vi "testAggState.vi"(8 "error in (no error)":errorcluster) -> (0 "error out":errorcluster)   [LabVIEW 2016]
doc: "Test the aggState.vi."
uses:
  ZTAAC/ZTAAC.lvclass
  StrictDef/DofGroup.ctl
  StrictDef/InstName.ctl
  <vilib>/addons/_JKI Toolkits/Caraya/classes/Test/Test.lvclass
  <vilib>/addons/_JKI Toolkits/Caraya/classes/Assert/Assert.lvclass
panel:
  in  "ZTAAC.lvclass":refnum<class "ZTAAC.lvclass">
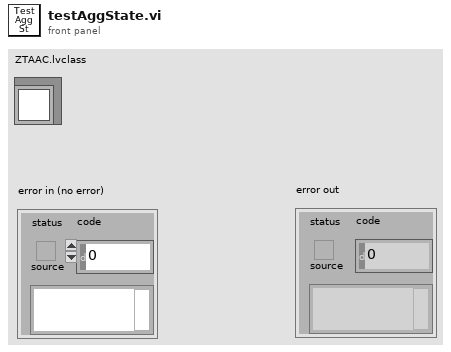
[diagram p1: front panel]
types:
  T1 = typedef "InstName.ctl" = enum16{"lsst", "comcam"}
  T2 = cluster{"Config Dir":path, "Inst Name":T1, "OptStateEsti Config File Name":string, "Mapping File Name":string, "Wavelength Table":string, "Intrinc Zk File Name":string, "y2 Corection File Name":string, "Index DOF File Name":string, "OptCtrl Config File Name":string, "State 0 File Name":string, "Weighting File Name":string, "PSSN Alpha File Name":string, "Authority Files":cluster{"Rigid Body Stroke File":string, "M1M3 Subsystem":cluster{"Mirror":string, "Actuatro Force File":string}, "M2 Subsystem":cluster{"Mirror":string, "Actuatro Force File":string}, "Num of Bending Mode":i32}, "Truncation Threshold":dbl}
  T3 = typedef "DofGroup.ctl" = enum16{"M2 Hex Pos", "Cam Hex Pos", "M1M3 Bend", "M2 Bend"}
  T4 = cluster{"M2 Hexapod":bool[], "Cam Hexapod ":bool[], "M1M3 Bending Mode":bool[], "M2 Bending Mode":bool[]}
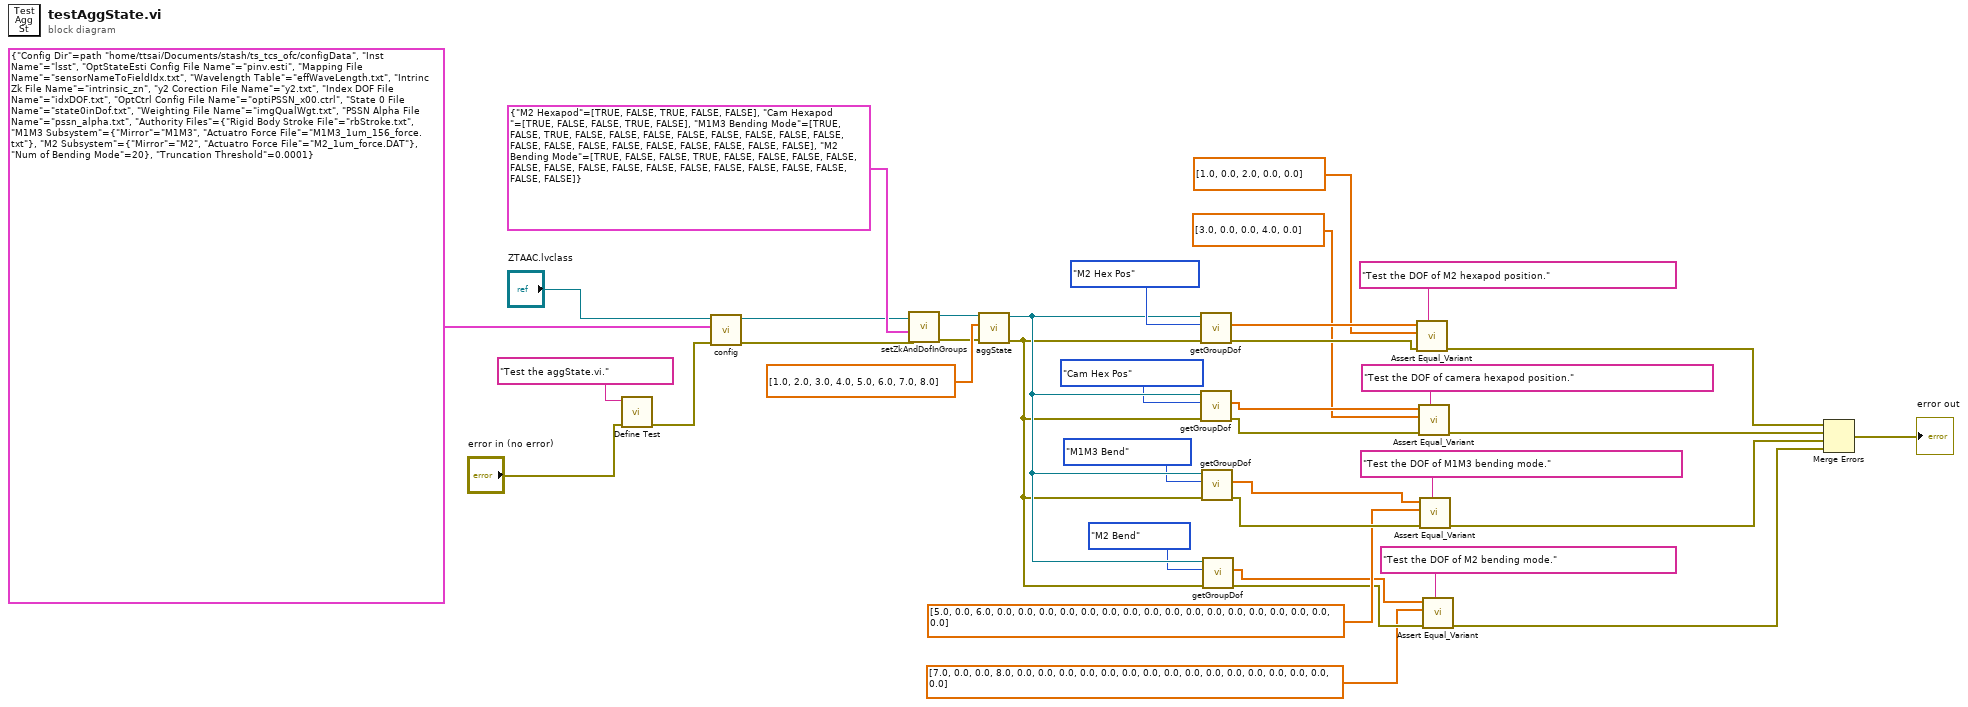
[diagram p0: block diagram]
diagram:
  n1 = call <vilib>:"Define Test.vi"("error in (no error)"="error in (no error)", "Label (VI Title)"="Test the aggState.vi.") -> ("error out"=w28:errorcluster)  [unwired: 9 in]
  n2 = call "config.vi"("error in (no error)"=w28, "ZTAAC Configuration"=T2 {"Config Dir"=path "/home/ttsai/Documents/stash/ts_tcs_ofc/configData", "Inst Name"=enum."lsst", "OptStateEsti Config File Name"="pinv.esti", "Mapping File Name"="sensorNameToFieldIdx.txt", "Wavelength Table"="effWaveLength.txt", "Intrinc Zk File Name"="intrinsic_zn", "y2 Corection File Name"="y2.txt", "Index DOF File Name"="idxDOF.txt", "OptCtrl Config File Name"="optiPSSN_x00.ctrl", "State 0 File Name"="state0inDof.txt", "Weighting File Name"="imgQualWgt.txt", "PSSN Alpha File Name"="pssn_alpha.txt", "Authority Files"={"Rigid Body Stroke File"="rbStroke.txt", "M1M3 Subsystem"={"Mirror"="M1M3", "Actuatro Force File"="M1M3_1um_156_force.txt"}, "M2 Subsystem"={"Mirror"="M2", "Actuatro Force File"="M2_1um_force.DAT"}, "Num of Bending Mode"=20}, "Truncation Threshold"=0.0001}, "ZTAAC in"="ZTAAC.lvclass") -> ("error out"=w25:errorcluster, "ZTAAC out"=w33:refnum<class "ZTAAC.lvclass">)  [unwired: 7 in]
  n3 = call "setZkAndDofInGroups.vi"("error in (no error)"=w25, "DOF in Groups"=T4 {"M2 Hexapod"=[TRUE, FALSE, TRUE, FALSE, FALSE], "Cam Hexapod "=[TRUE, FALSE, FALSE, TRUE, FALSE], "M1M3 Bending Mode"=[TRUE, FALSE, TRUE, FALSE, FALSE, FALSE, FALSE, FALSE, FALSE, FALSE, FALSE, FALSE, FALSE, FALSE, FALSE, FALSE, FALSE, FALSE, FALSE, FALSE], "M2 Bending Mode"=[TRUE, FALSE, FALSE, TRUE, FALSE, FALSE, FALSE, FALSE, FALSE, FALSE, FALSE, FALSE, FALSE, FALSE, FALSE, FALSE, FALSE, FALSE, FALSE, FALSE]}, "ZTAAC in"=w33) -> ("error out"=w24:errorcluster, "ZTAAC out"=w36:refnum<class "ZTAAC.lvclass">)  [unwired: 7 in]
  n4 = call "aggState.vi"("error in (no error)"=w24, "State in DOF"=dbl[] [1.0, 2.0, 3.0, 4.0, 5.0, 6.0, 7.0, 8.0], "ZTAAC in"=w36) -> ("error out"=w23:errorcluster, "ZTAAC out"=w32:refnum<class "ZTAAC.lvclass">)  [unwired: 7 in]
  n5 = call "getGroupDof.vi"("error in (no error)"=w23, "DOF Group"=DofGroup."M2 Hex Pos", "ZTAAC in"=w32) -> ("error out"=w21:errorcluster, "DOF"=w22:dbl[])  [unwired: 6 in, 1 out]
  n6 = call "getGroupDof.vi"("error in (no error)"=w23, "DOF Group"=DofGroup."Cam Hex Pos", "ZTAAC in"=w32) -> ("error out"=w14:errorcluster, "DOF"=w13:dbl[])  [unwired: 6 in, 1 out]
  n7 = call "getGroupDof.vi"("error in (no error)"=w23, "DOF Group"=DofGroup."M1M3 Bend", "ZTAAC in"=w32) -> ("error out"=w9:errorcluster, "DOF"=w8:dbl[])  [unwired: 6 in, 1 out]
  n8 = call "getGroupDof.vi"("error in (no error)"=w23, "DOF Group"=DofGroup."M2 Bend", "ZTAAC in"=w32) -> ("error out"=w5:errorcluster, "DOF"=w4:dbl[])  [unwired: 6 in, 1 out]
  n9 = call <vilib>:"Assert Equal_Variant.vi"("Label"="Test the DOF of M2 hexapod position.", "error in (no error)"=w21, "Y"=dbl[] [1.0, 0.0, 2.0, 0.0, 0.0] ("State in DOF"), "X"=w22) -> ("error out"=w17:errorcluster)  [unwired: 7 in]
  n10 = call <vilib>:"Assert Equal_Variant.vi"("Label"="Test the DOF of camera hexapod position.", "error in (no error)"=w14, "Y"=dbl[] [3.0, 0.0, 0.0, 4.0, 0.0] ("State in DOF"), "X"=w13) -> ("error out"=w16:errorcluster)  [unwired: 7 in]
  n11 = call <vilib>:"Assert Equal_Variant.vi"("Label"="Test the DOF of M1M3 bending mode.", "error in (no error)"=w9, "Y"=dbl[] [5.0, 0.0, 6.0, 0.0, 0.0, 0.0, 0.0, 0.0, 0.0, 0.0, 0.0, 0.0, 0.0, 0.0, 0.0, 0.0, 0.0, 0.0, 0.0, 0.0] ("State in DOF"), "X"=w8) -> ("error out"=w10:errorcluster)  [unwired: 7 in]
  n12 = call <vilib>:"Assert Equal_Variant.vi"("Label"="Test the DOF of M2 bending mode.", "error in (no error)"=w5, "Y"=dbl[] [7.0, 0.0, 0.0, 8.0, 0.0, 0.0, 0.0, 0.0, 0.0, 0.0, 0.0, 0.0, 0.0, 0.0, 0.0, 0.0, 0.0, 0.0, 0.0, 0.0] ("State in DOF"), "X"=w4) -> ("error out"=w3:errorcluster)  [unwired: 7 in]
  n13 = Merge Errors(w17, w16, w10, w3) -> (→"error out":errorcluster)
